vi "GetParam.vi"(8 "error in (no error)":errorcluster caption="entrée d'erreur (pas d'erreur)", 11 "RepeatedKFold.lvclass":refnum<class "RepeatedKFold.lvclass">) -> (0 "error out":errorcluster caption="sortie d'erreur", 2 "RepeatedKFold":T1={"n_splits"=5, "n_repeats"=10, "random_state"=-1} {"random_state" min=-1}, 3 "RepeatedKFold.lvclass":refnum<class "RepeatedKFold.lvclass">)   [LabVIEW 2020, in "RepeatedKFold.lvclass"]
doc: "Get Parameters"
uses:
  RepeatedKFold.lvclass
  RepeatedKFold.lvclass/RepeatedKFold.ctl
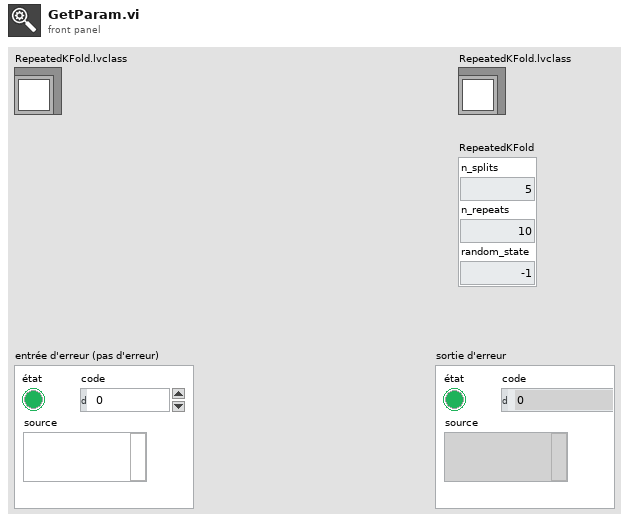
[diagram p1: front panel]
types:
  T1 = cluster{"n_splits":i32, "n_repeats":i32, "random_state":i32}
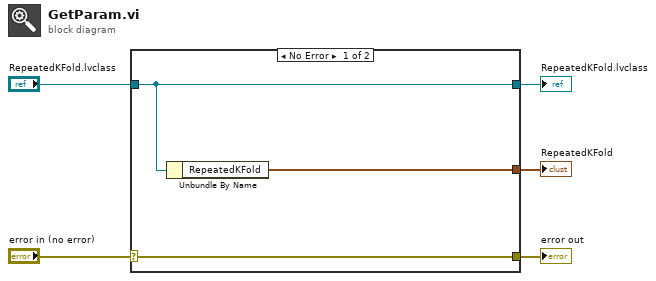
[diagram p0: block diagram]
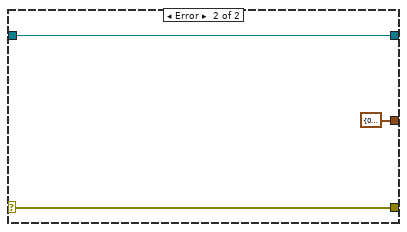
[diagram p2: hidden frame]
diagram:
  n1 = case shown="No Error" "error in (no error)" {
    selector: "error in (no error)" -> [w8 w10]
    tunnel: [w8 w10] -> w4
    tunnel: [w7 w11] -> w2
    tunnel: "RepeatedKFold.lvclass" -> [w7 w11]
    tunnel: [w6 T1 {"n_splits"=0, "n_repeats"=0, "random_state"=0} ("RepeatedKFold")] -> w1
    frame No Error {
      n2 = Unbundle By Name(w7) -> ("RepeatedKFold"=w6:T1)
    }
    frame Error {
    }
  }
  "error out" <- w4
  "RepeatedKFold.lvclass" <- w2
  "RepeatedKFold" <- w1
